vi "SubVI_makeLabelLeftCenter.vi"(8 "error in":errorcluster, 11 "Refnum in":refnum<vi>) -> (0 "error out":errorcluster, 3 "Refnum out":refnum<vi>)   [LabVIEW 2015]
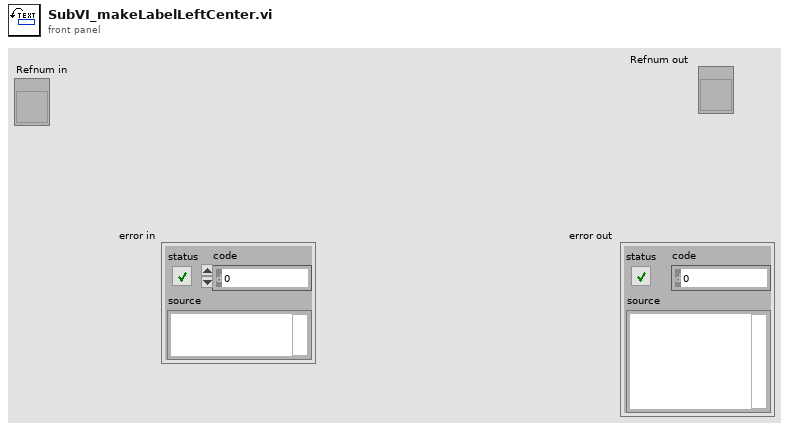
[diagram p1: front panel]
types:
  T1 = typedef "LVPositionTypeDef.ctl" = cluster{"Left":i32, "Top":i32}
  T2 = typedef "LVBoundsTypeDef.ctl" = cluster{"Width":u32, "Height":u32}
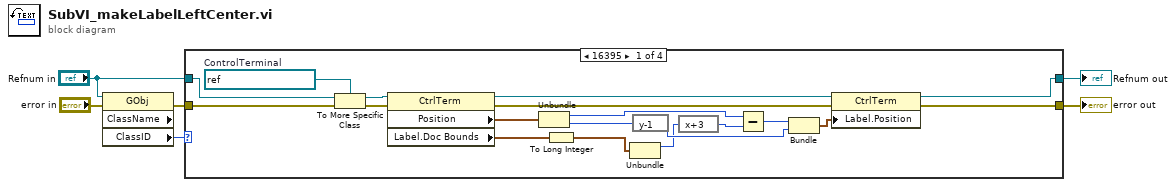
[diagram p0: block diagram]
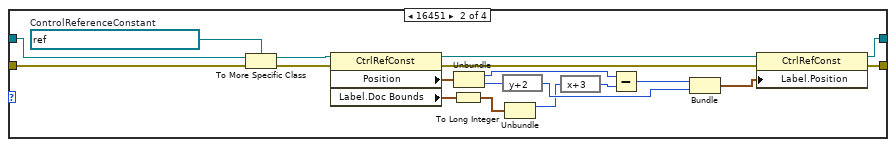
[diagram p2: hidden frame]
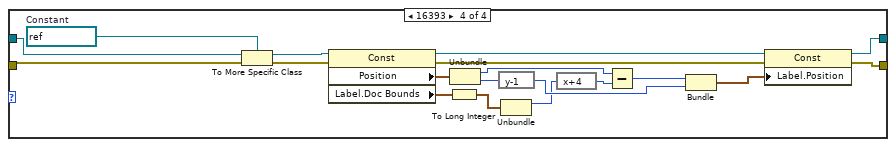
[diagram p4: hidden frame]
diagram:
  n1 = property on="Property Node" class="GObj" props=["ClassName", "ClassID"](reference="Refnum in", error in="error in") -> (error out=w3:errorcluster, "ClassID"=w4:u32)  [unwired: 2 out]
  n2 = case shown="16395" w4 {
    tunnel: w3 -> [w11 w44 w45 w49]
    tunnel: "Refnum in" -> [w12 w43 w46 w50]
    tunnel: [w10 w42 w46 w48] -> w5
    tunnel: [w9 w41 w45 w47] -> w6
    frame 16395 {
      w25 = refnum<vi> refnum  # ControlTerminal
      n3 = To More Specific Class(target class=w25, reference=w12, error in=w11) -> (specific class reference=w8:refnum<vi>, error out=w7:errorcluster)
      n4 = property on="Property Node" class="CtrlTerm"(reference=w8, error in=w7) -> (reference out=w24:refnum<vi>, error out=w15:errorcluster, "Position"=w23:T1, "Label.Doc Bounds"=w14:T2)
      n5 = Unbundle(w23) -> ("Left"=w18:i32, "Top"=w20:i32)
      n6 = To Long Integer(number=w14) -> (32bit integer=w13:cluster{"Width":i32, "Height":i32})
      n7 = Unbundle(w13) -> ("Width"=w19:i32)  [unwired: 1 out]
      n8 = expression code="y-1"(w20) -> (w21:i32)
      n9 = expression code="x+3"(w19) -> (w17:i32)
      n10 = Subtract(x=w18, y=w17) -> (x-y=w16:i32)
      n11 = Bundle(w16, "Top"=w21) -> (w22:cluster{i32, "Top":i32})  [unwired: 1 in]
      n12 = property on="Property Node" class="CtrlTerm"(reference=w24, error in=w15, "Label.Position"=w22) -> (reference out=w10:refnum<vi>, error out=w9:errorcluster)
    }
    frame 16451 {
      w40 = refnum<vi> refnum  # ControlReferenceConstant
      n13 = To More Specific Class(target class=w40, reference=w43, error in=w44) -> (specific class reference=w39:refnum<vi>, error out=w38:errorcluster)
      n14 = property on="Property Node" class="CtrlRefConst"(reference=w39, error in=w38) -> (reference out=w37:refnum<vi>, error out=w28:errorcluster, "Position"=w36:T1, "Label.Doc Bounds"=w27:T2)
      n15 = To Long Integer(number=w27) -> (32bit integer=w26:cluster{"Width":i32, "Height":i32})
      n16 = Unbundle(w36) -> ("Left"=w31:i32, "Top"=w33:i32)
      n17 = expression code="y+2"(w33) -> (w34:i32)
      n18 = Unbundle(w26) -> ("Width"=w32:i32)  [unwired: 1 out]
      n19 = expression code="x+3"(w32) -> (w30:i32)
      n20 = Subtract(x=w31, y=w30) -> (x-y=w29:i32)
      n21 = Bundle(w29, "Top"=w34) -> (w35:cluster{i32, "Top":i32})  [unwired: 1 in]
      n22 = property on="Property Node" class="CtrlRefConst"(reference=w37, error in=w28, "Label.Position"=w35) -> (reference out=w42:refnum<vi>, error out=w41:errorcluster)
    }
    frame Default {
    }
    frame 16393 {
      w65 = refnum<vi> refnum  # Constant
      n23 = To More Specific Class(target class=w65, reference=w50, error in=w49) -> (specific class reference=w64:refnum<vi>, error out=w63:errorcluster)
      n24 = property on="Property Node" class="Const"(reference=w64, error in=w63) -> (reference out=w62:refnum<vi>, error out=w53:errorcluster, "Position"=w61:T1, "Label.Doc Bounds"=w52:T2)
      n25 = To Long Integer(number=w52) -> (32bit integer=w51:cluster{"Width":i32, "Height":i32})
      n26 = Unbundle(w61) -> ("Left"=w56:i32, "Top"=w58:i32)
      n27 = expression code="y-1"(w58) -> (w59:i32)
      n28 = Unbundle(w51) -> ("Width"=w57:i32)  [unwired: 1 out]
      n29 = expression code="x+4"(w57) -> (w55:i32)
      n30 = Subtract(x=w56, y=w55) -> (x-y=w54:i32)
      n31 = Bundle(w54, "Top"=w59) -> (w60:cluster{i32, "Top":i32})  [unwired: 1 in]
      n32 = property on="Property Node" class="Const"(reference=w62, error in=w53, "Label.Position"=w60) -> (reference out=w48:refnum<vi>, error out=w47:errorcluster)
    }
  }
  "error out" <- w6
  "Refnum out" <- w5
